vi "实验2_1.vi"() -> ()   [LabVIEW 2018]
panel:
  in  "k":dbl=2.0
  in  "var":dbl=1.0
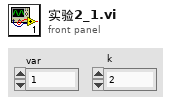
[diagram p1: front panel]
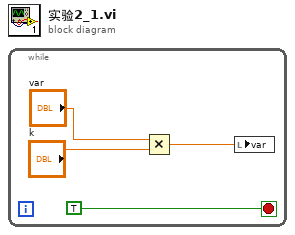
[diagram p0: block diagram]
diagram:
  n1 = while {
    stop <- TRUE stop-if-true
    n2 = Multiply(x="var", y="k") -> (x*y=w4:dbl)
    n3 = local write "var"(w4) -> ()
  }
